vi "PH_Cont-601k_PowerUnit.Switch SM.vi"(0 "VI in":refnum<vi>, 5 "error in (no error)":errorcluster) -> (14 "VI out":refnum<vi>, 19 "error out":errorcluster)   [LabVIEW 2014, in "PH_Cont-601k_PowerUnit.lvlib"]
uses:
  PH_Cont-601k_PowerUnit.lvlib
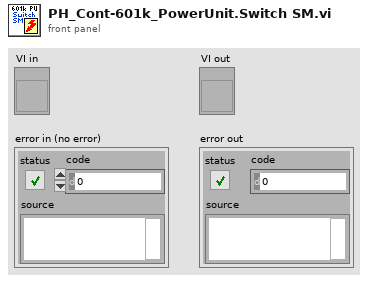
[diagram p1: front panel]
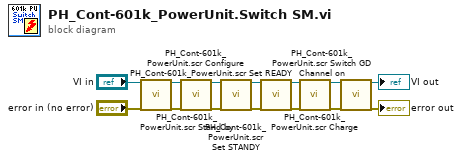
[diagram p0: block diagram]
diagram:
  n1 = call "PH_Cont-601k_PowerUnit.scr Stand by.vi"("VI in"="VI in", "error in (no error)"="error in (no error)") -> ("VI out"=w12:refnum<vi>, "error out"=w11:errorcluster)  [unwired: 16 in]
  n2 = call "PH_Cont-601k_PowerUnit.scr Configure.vi"("VI in"=w12, "error in (no error)"=w11) -> ("VI out"=w14:refnum<vi>, "error out"=w13:errorcluster)  [unwired: 16 in]
  n3 = call "PH_Cont-601k_PowerUnit.scr Set STANDY.vi"("VI in"=w14, "error in (no error)"=w13) -> ("VI out"=w9:refnum<vi>, "error out"=w10:errorcluster)  [unwired: 16 in]
  n4 = call "PH_Cont-601k_PowerUnit.scr Set READY.vi"("VI in"=w9, "error in (no error)"=w10) -> ("VI out"=w4:refnum<vi>, "error out"=w3:errorcluster)  [unwired: 16 in]
  n5 = call "PH_Cont-601k_PowerUnit.scr Charge.vi"("VI in"=w4, "error in (no error)"=w3) -> ("VI out"=w6:refnum<vi>, "error out"=w5:errorcluster)  [unwired: 16 in]
  n6 = call "PH_Cont-601k_PowerUnit.scr Switch GD Channel on.vi"("VI in"=w6, "error in (no error)"=w5) -> ("VI out"=→"VI out":refnum<vi>, "error out"=→"error out":errorcluster)  [unwired: 16 in]
